vi "ALTS-2015 Check Serial Number before Starting Test.vi"(8 "error in (no error)":errorcluster, 10 "Station Details":T1={"Station Number"="", "Work Order Number"="", "Sensor Name"="", "Pressure (PSI)"="", "Flow (SCCM)"="", "Test Time "="", "Test Result"="", "Serial Number"="", "Station Status"=0, "SW assigned UUT"=FALSE, "Rerun Count"=0, "Test Type"=0, "Load Decision"=0, "Robot Action"=enum."No Action"}) -> (0 "error out":errorcluster, 2 "Station Details Out":T1={"Station Number"="", "Work Order Number"="", "Sensor Name"="", "Pressure (PSI)"="", "Flow (SCCM)"="", "Test Time "="", "Test Result"="", "Serial Number"="", "Station Status"=0, "SW assigned UUT"=FALSE, "Rerun Count"=0, "Test Type"=0, "Load Decision"=0, "Robot Action"=enum."No Action"}, 3 "SN Empty?":bool)   [LabVIEW 2013]
doc: "Copyright © 2005, Soliton Technologies.\nAll rights reserved."
uses:
  Controls/ALTS-2015 Station Details.ctl
  Controls/ALTS-2015 Status Ring Indicator.ctl
  Controls/ALTS-2015 Robot Actions.ctl
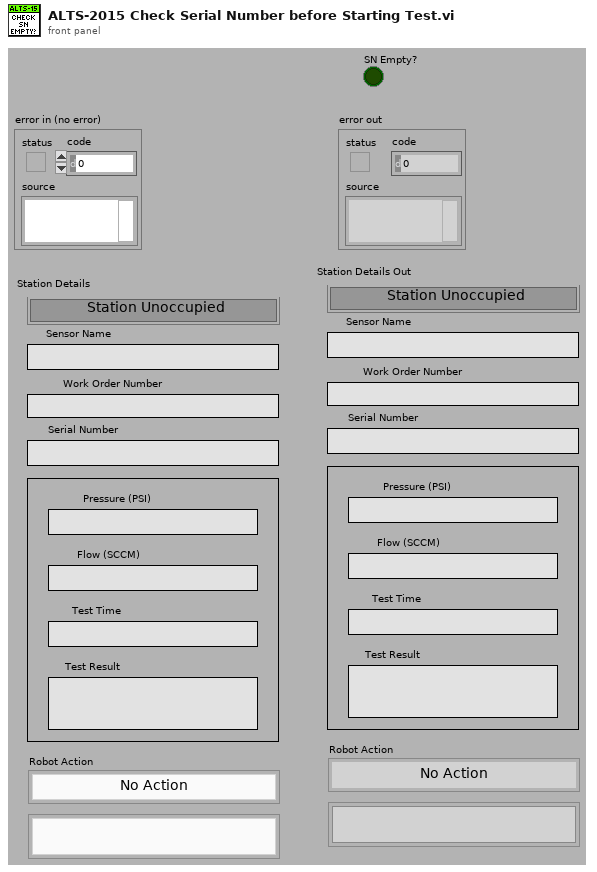
[diagram p1: front panel]
types:
  T1 = typedef "ALTS-2015 Station Details.ctl" = cluster{"Station Number":string, "Work Order Number":string, "Sensor Name":string, "Pressure (PSI)":string, "Flow (SCCM)":string, "Test Time ":string, "Test Result":string, "Serial Number":string, "Station Status":T2, "SW assigned UUT":bool, "Rerun Count":i32, "Test Type":i32, "Load Decision":i32, "Robot Action":T3}
  T2 = typedef "ALTS-2015 Status Ring Indicator.ctl" = u16
  T3 = typedef "ALTS-2015 Robot Actions.ctl" = enum16{"Loading...", "Unloading...", "Reruning...", "No Action"}
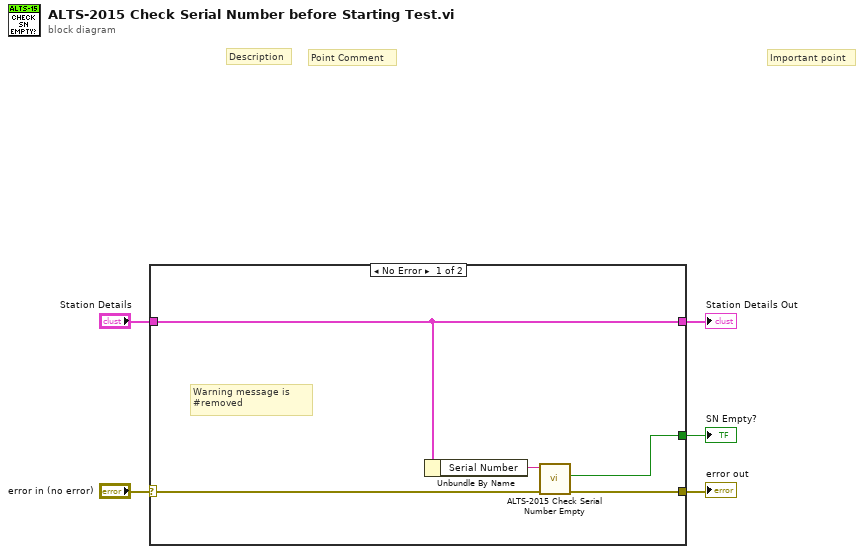
[diagram p0: block diagram]
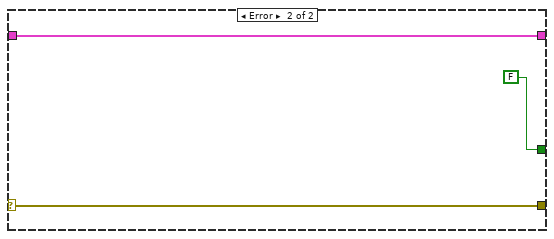
[diagram p2: hidden frame]
diagram:
  # "Point Comment"
  # "Important point"
  # "Description"
  n1 = case shown="No Error" "error in (no error)" {
    selector: "error in (no error)" -> [w9 w13]
    tunnel: [w8 w13] -> w4
    tunnel: "Station Details" -> [w7 w12]
    tunnel: [w7 w12] -> w2
    tunnel: [w6 FALSE ("SN Empty?")] -> w1
    frame No Error {
      # "Warning message is \n#removed"
      n2 = Unbundle By Name(w7) -> ("Serial Number"=w10:string)
      n3 = call "ALTS-2015 Check Serial Number Empty.vi"("error in (no error)"=w9, "Serial Number"=w10) -> ("error out"=w8:errorcluster, "SN Empty?"=w6:bool)  [unwired: 7 in, 1 out]
    }
    frame Error {
    }
  }
  "error out" <- w4
  "Station Details Out" <- w2
  "SN Empty?" <- w1
